vi "MT Generate QAM System Parameters(M).vi"(0 "samples per symbol (16)":i32=16, 5 "M-QAM (16)":i32=16, 11 "error in (no error)":errorcluster) -> (6 "QAM system parameters":T1 {"symbol map" format="%.3f"}, 8 "bits per symbol":i32, 15 "error out":errorcluster)   [LabVIEW 2020, in "niDMT.lvlib"]
doc: "This polymorphic instance calculates parameters for use with either the MT Modulate QAM VI or the MT Demodulate QAM VI. It accepts an M-ary value that specifies a predefined symbol map with the number of distinct symbol map values to use as symbols."
uses:
  <vilib>/addons/Modulation/niDMT.lvlib
  <vilib>/addons/Modulation/Digital/Support/Controls/QAM System Parameters.ctl
  <vilib>/addons/Modulation/niAMT.lvlib
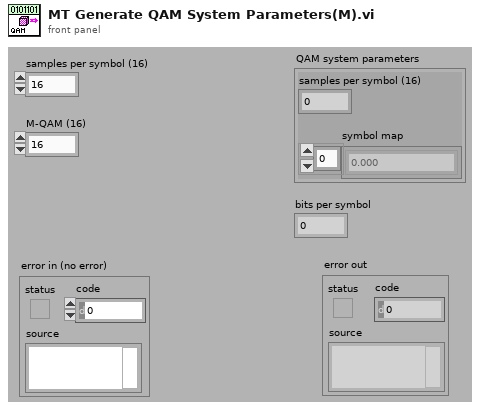
[diagram p1: front panel]
types:
  T1 = cluster{"samples per symbol (16)":i32, "symbol map":cdb[]}
  T2 = typedef "niDMT.lvlib/QAM System Parameters.ctl" = cluster{"samples per symbol (16)":i32, "symbol map":cdb[]}
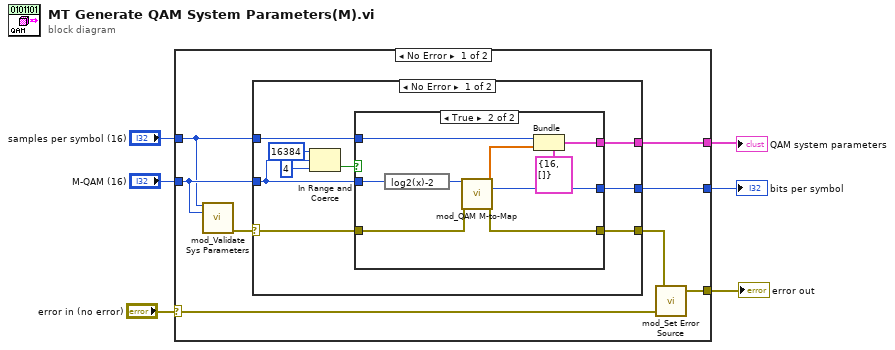
[diagram p0: block diagram]
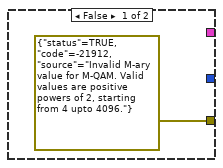
[diagram p2: hidden frame]
diagram:
  n1 = case shown="No Error" "error in (no error)" {
    selector: "error in (no error)" -> [w10 w35]
    tunnel: "samples per symbol (16)" -> [w7 _]
    tunnel: [w14 _] -> w5
    tunnel: [w11 _] -> w4
    tunnel: [w13 w35] -> w3
    tunnel: "M-QAM (16)" -> [w8 _]
    frame No Error {
      n2 = call <vilib>:"mod_Validate Sys Parameters.vi"("samples per symbol"=w7, "M-ary"=w8) -> ("error out"=w9:errorcluster)  [unwired: 13 out]
      n3 = case shown="No Error" w9 {
        selector: w9 -> [w19 w34]
        tunnel: [w23 _] -> w14
        tunnel: [w22 w34] -> w12
        tunnel: [w21 _] -> w11
        tunnel: w8 -> [w17 _]
        tunnel: w7 -> [w20 _]
        frame No Error {
          n4 = In Range and Coerce(upper limit=16384 ("lower limit"), x=w17, lower limit=4 ("upper limit")) -> (In Range?=w18:bool)  [unwired: 1 out]
          n5 = case shown="True" w18 {
            tunnel: [_ w33] -> w23
            tunnel: [errorcluster {"status"=TRUE, "code"=-21912, "source"="Invalid M-ary value for M-QAM. Valid values are positive powers of 2, starting from 4 upto 4096."} ("error out") w31] -> w22
            tunnel: [_ w30] -> w21
            tunnel: w17 -> [_ w26]
            tunnel: w20 -> [_ w28]
            tunnel: w19 -> [_ w29]
            frame False {
            }
            frame True {
              n6 = expression code="log2(x)-2"(w26) -> (w25:i32)
              n7 = call <vilib>:"mod_QAM M-to-Map.vi"("M selection"=w25, "error in (no error)"=w29) -> ("Symbol Map"=w32:cdb[], "bits/symbol"=w30:i32, "error out"=w31:errorcluster)  [unwired: 11 out]
              n8 = Bundle(cluster=T2 {"samples per symbol (16)"=16, "symbol map"=[]} ("QAM system parameters"), "samples per symbol (16)"=w28, "symbol map"=w32) -> (w33:T2)
            }
          }
        }
        frame Error {
        }
      }
      n9 = call <vilib>:"mod_Set Error Source.vi"("initial error in (no error)"=w10, "final error in (no error)"=w12) -> ("error out"=w13:errorcluster)  [unwired: 3 out]
    }
    frame Error {
    }
  }
  "QAM system parameters" <- w5
  "bits per symbol" <- w4
  "error out" <- w3
